vi "arrayTransparent.vi"() -> ()   [LabVIEW 2020]
panel:
  in  "White Array":cluster{"String":string, "String 2":string}[](array[cluster])
  in  "Transparent Array":cluster{"String":string, "String 2":string}[](array[cluster])
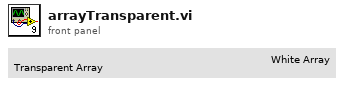
[diagram p1: front panel]
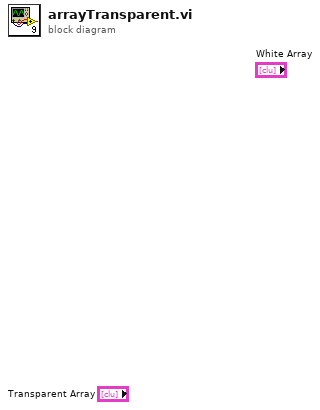
[diagram p0: block diagram]
diagram:
